vi "Write Switch File Info.vi"(10 "Switch File Info":string, 11 "SLSC Switch in":refnum<class "SLSC Switch.lvclass">) -> (3 "SLSC Switch out":refnum<class "SLSC Switch.lvclass">)   [LabVIEW 2015, in "SLSC Switch.lvclass"]
uses:
  SLSC Switch.lvclass
  SLSC Switch.lvclass/SLSC Switch.ctl
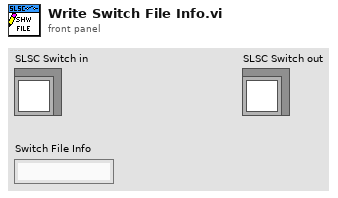
[diagram p1: front panel]
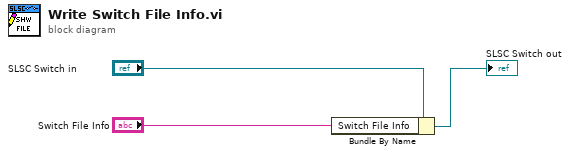
[diagram p0: block diagram]
diagram:
  n1 = Bundle By Name(cluster="SLSC Switch in", "Switch File Info"="Switch File Info") -> (→"SLSC Switch out":refnum<class "SLSC Switch.lvclass">)
